vi "Driving with the Limelight search and aim.vi"(8 "error in (no error)":errorcluster) -> (0 "TurnCommand":dbl(knob)=nan scale=-1.0..1.0, 1 "SpeedCommand":dbl(knob)=-0.0 scale=0.0..1.0, 3 "TargetValid":bool)   [LabVIEW 2019]
uses:
  Framework/Robot Global Data.vi
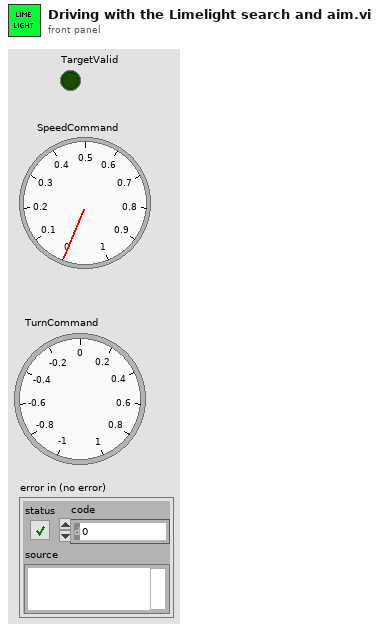
[diagram p1: front panel]
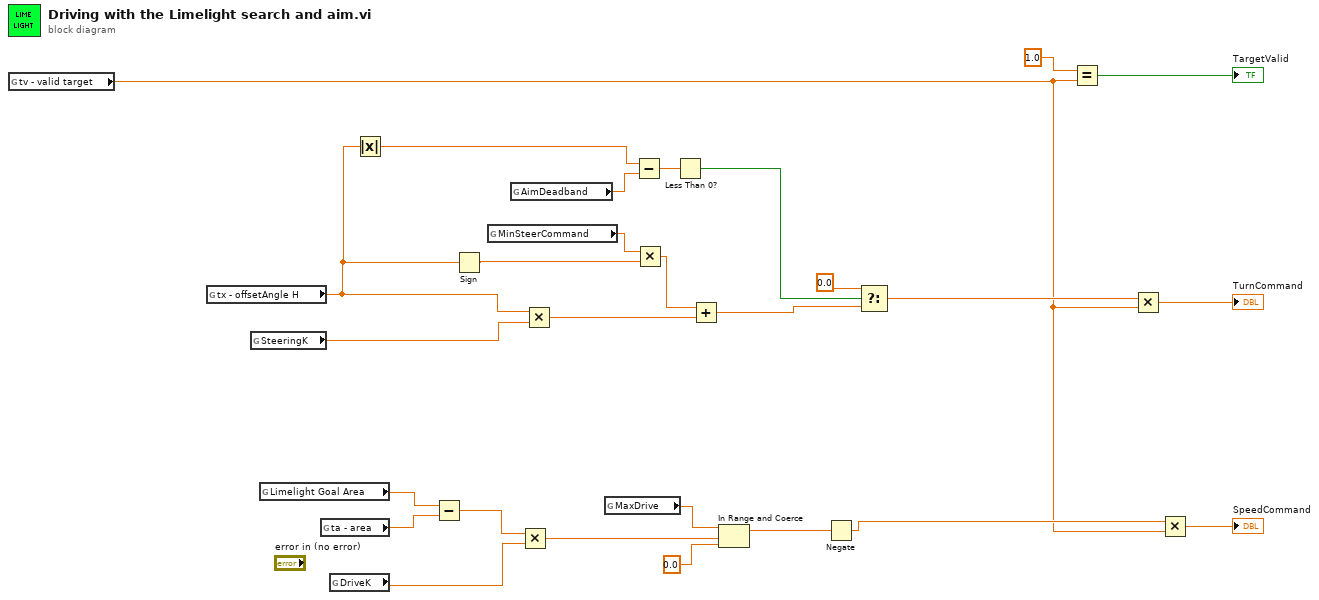
[diagram p0: block diagram]
diagram:
  n1 = global read "Robot Global Data.vi" "tv - valid target"() -> (w1:dbl)
  n2 = global read "Robot Global Data.vi" "tx - offsetAngle H"() -> (w12:dbl)
  n3 = global read "Robot Global Data.vi" "SteeringK"() -> (w7:dbl)
  n4 = global read "Robot Global Data.vi" "Limelight Goal Area"() -> (w8:dbl)
  n5 = global read "Robot Global Data.vi" "ta - area"() -> (w11:dbl)
  n6 = global read "Robot Global Data.vi" "DriveK"() -> (w9:dbl)
  n7 = Absolute Value(x=w12) -> (abs(x)=w21:dbl)
  n8 = Subtract(x=w8, y=w11) -> (x-y=w17:dbl)
  n9 = Sign(1:w12) -> (0:w18:dbl)
  n10 = global read "Robot Global Data.vi" "MinSteerCommand"() -> (w5:dbl)
  n11 = global read "Robot Global Data.vi" "AimDeadband"() -> (w6:dbl)
  n12 = Multiply(x=w17, y=w9) -> (x*y=w16:dbl)
  n13 = Multiply(x=w12, y=w7) -> (x*y=w19:dbl)
  n14 = global read "Robot Global Data.vi" "MaxDrive"() -> (w10:dbl)
  n15 = Subtract(x=w21, y=w6) -> (x-y=w22:dbl)
  n16 = Multiply(x=w5, y=w18) -> (x*y=w20:dbl)
  n17 = Less Than 0?(x=w22) -> (x < 0?=w23:bool)
  n18 = Add(x=w20, y=w19) -> (x+y=w4:dbl)
  n19 = In Range and Coerce(upper limit=w10, x=w16, lower limit=0.0) -> (coerced(x)=w14:dbl)  [unwired: 1 out]
  n20 = Negate(x=w14) -> (-x=w27:dbl)
  n21 = Select(t=0.0, s=w23, f=w4) -> (s? t:f=w25:dbl)
  n22 = Equal?(x=1.0, y=w1) -> (x = y?=→"TargetValid":bool)
  n23 = Multiply(x=w25, y=w1) -> (x*y=→"TurnCommand":dbl)
  n24 = Multiply(x=w27, y=w1) -> (x*y=→"SpeedCommand":dbl)
